vi "油动机0%和100%位置.vi"(4 "计算参数 in":T2, 5 "输入参数 in":T1, 7 "Array in":dbl[](array[numeric])) -> (0 "计算参数 out":T2, 1 "输入参数 out":T1, 3 "Array out":dbl[](array[numeric]))   [LabVIEW 2013]
doc: "计算灵敏度Sen，以及油动机处在打开和关闭状态时对应的电流值\n【灵敏度Sen】Sen（mA/mm）=（100%mA－0%mA）∕Gh。Gh为手工输入。\n【V1】Ｖ1（mA）＝0%mA＋Sen×Oh1\n【V2】Ｖ2（mA）＝0%mA＋Sen×（Oh1+Ah）"
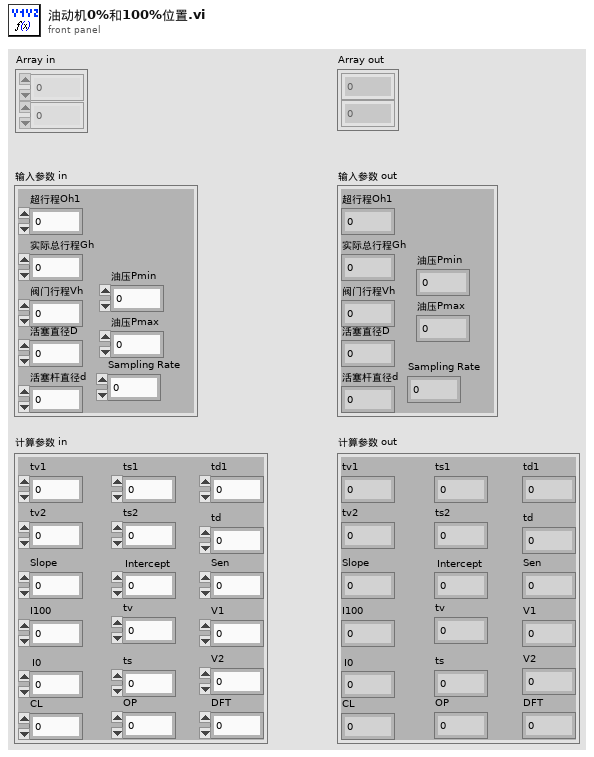
[diagram p1: front panel]
types:
  T1 = cluster{"超行程Oh1":dbl, "实际总行程Gh":dbl, "阀门行程Vh":dbl, "活塞直径D":dbl, "活塞杆直径d":dbl, "油压Pmin":dbl, "油压Pmax":dbl, "Sampling Rate":dbl}
  T2 = cluster{"tv1":dbl, "tv2":dbl, "tv":dbl, "ts1":dbl, "ts2":dbl, "ts":dbl, "td1":dbl, "td":dbl, "Slope":dbl, "Intercept":dbl, "I100":dbl, "I0":dbl, "Sen":dbl, "V1":dbl, "V2":dbl, "CL":dbl, "OP":dbl, "DFT":dbl}
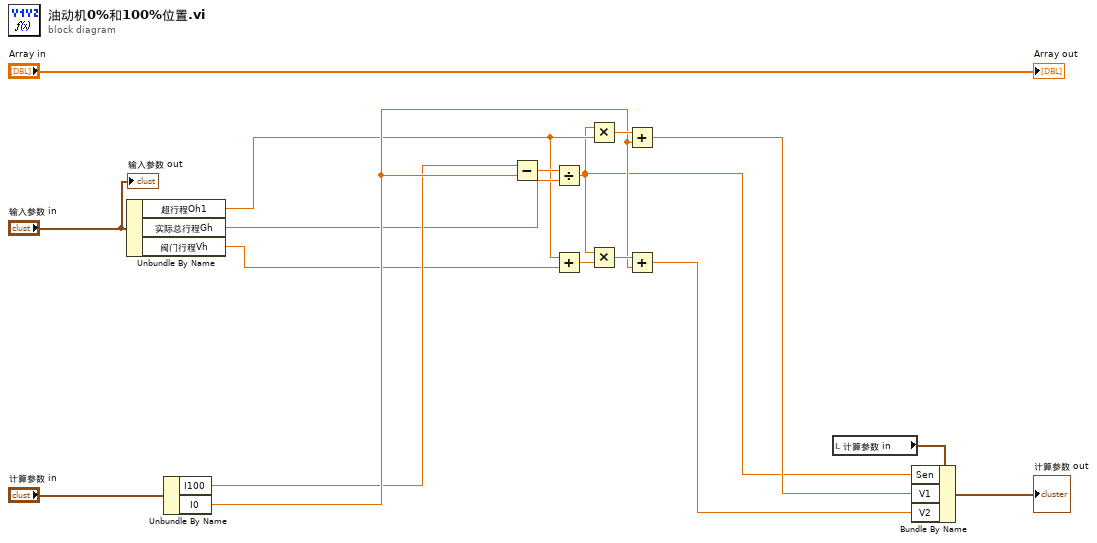
[diagram p0: block diagram]
diagram:
  n1 = Unbundle By Name("输入参数 in") -> ("超行程Oh1"=w7:dbl, "实际总行程Gh"=w8:dbl, "阀门行程Vh"=w6:dbl)
  n2 = Unbundle By Name("计算参数 in") -> ("I100"=w9:dbl, "I0"=w10:dbl)
  n3 = Subtract(x=w9, y=w10) -> (x-y=w14:dbl)
  n4 = Divide(x=w14, y=w8) -> (x/y=w3:dbl)
  n5 = Add(x=w7, y=w6) -> (x+y=w16:dbl)
  n6 = Multiply(x=w3, y=w7) -> (x*y=w15:dbl)
  n7 = Multiply(x=w3, y=w16) -> (x*y=w17:dbl)
  n8 = Add(x=w15, y=w10) -> (x+y=w5:dbl)
  n9 = Add(x=w17, y=w10) -> (x+y=w4:dbl)
  n10 = local read "计算参数 in"() -> (w11:T2)
  n11 = Bundle By Name(cluster=w11, "Sen"=w3, "V1"=w5, "V2"=w4) -> (→"计算参数 out":T2)
  "Array out" <- "Array in"
  "输入参数 out" <- "输入参数 in"
